vi "NPC3SG Live Control v10.6.2.vi"(1 "Running":refnum<vi>, 2 "Calibration File":path, 3 "Drive Live Controls":T1={"Snapshot"=FALSE, "Move Step"=0.5, "Move Home"=FALSE, "Move Down"=FALSE, "Move Up"=FALSE, "Move Left"=FALSE, "Move Right"=FALSE, "Move Out"=FALSE, "Move In"=FALSE} {"Move Step" min=0.0 max=30.0 step=0.1 format="%.3f"}, 4 "Drive Visa Name":refnum<visa-resource-name>="COM5") -> (0 "Reset Switches":bool)   [LabVIEW 2010]
uses:
  TypeDefs/NPC3SG Live Controls.ctl
panel:
  in  "Home":dbl=10.0 format="%.3f"
  # "XY"
  # "Z"
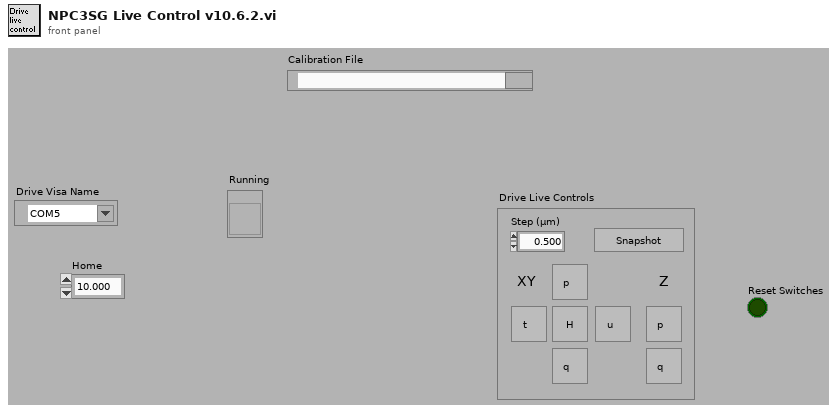
[diagram p1: front panel]
types:
  T1 = typedef "NPC3SG Live Controls.ctl" = cluster{"Snapshot":bool, "Move Step":dbl, "Move Home":bool, "Move Down":bool, "Move Up":bool, "Move Left":bool, "Move Right":bool, "Move Out":bool, "Move In":bool}
  T2 = typedef "NPC3SG Current Values.ctl" = cluster{"Drive X Position":dbl, "Drive Y Position":dbl, "Drive Z Position":dbl}
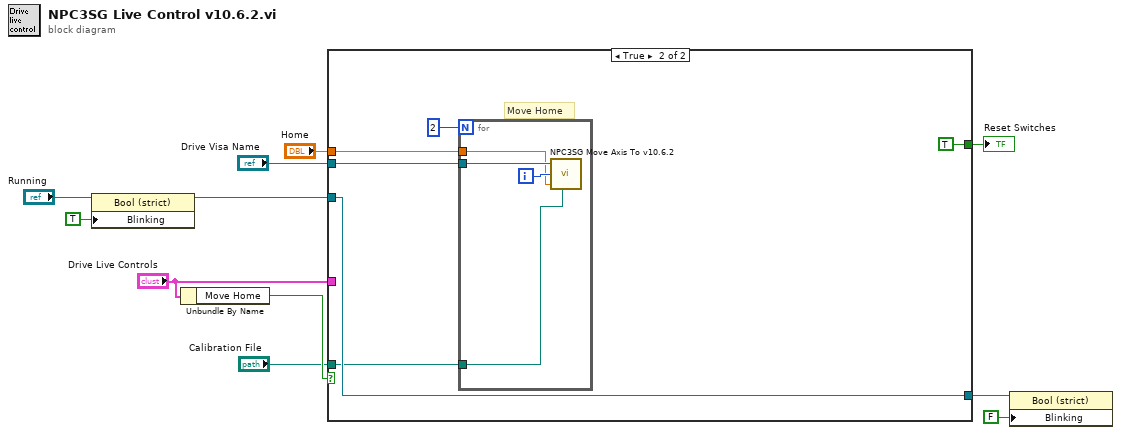
[diagram p0: block diagram]
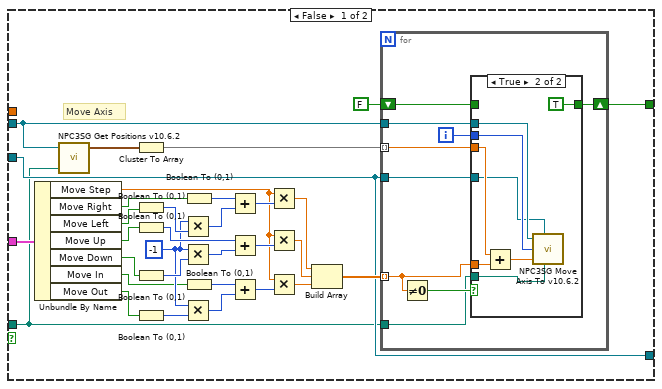
[diagram p2: hidden frame]
diagram:
  n1 = property class="Bool (strict)"(reference="Running", "Blinking"=TRUE ("Blinkend")) -> (reference out=w4:refnum<vi>)  [unwired: 1 in, 1 out]
  n2 = Unbundle By Name("Drive Live Controls") -> ("Move Home"=w9:bool)
  n3 = case shown="True" w9 {
    tunnel: "Drive Visa Name" -> [w18 w66]
    tunnel: [w16 TRUE ("Reset Switches")] -> w11
    tunnel: w4 -> [w14 w64]
    tunnel: "Drive Live Controls" -> [w19 _]
    tunnel: "Home" -> [_ w65]
    tunnel: [w14 w64] -> w2
    tunnel: "Calibration File" -> [w12 w62]
    frame False {
      w31 = -1
      # "Move Axis"
      n4 = Unbundle By Name(w19) -> ("Move Step"=w20:dbl, "Move Right"=w21:bool, "Move Left"=w26:bool, "Move Up"=w25:bool, "Move Down"=w24:bool, "Move In"=w23:bool, "Move Out"=w22:bool)
      n5 = call "NPC3SG Get Positions v10.6.2.vi"("Drive Visa Name"=w18, "Calibration File"=w12) -> ("Drive Current Values"=w13:T2)  [unwired: 5 in]
      n6 = Cluster To Array(cluster=w13) -> (array=w17:dbl[])
      n7 = Boolean To (0,1)(Boolean=w26) -> (0, 1=w33:i16)
      n8 = Boolean To (0,1)(Boolean=w25) -> (0, 1=w37:i16)
      n9 = Boolean To (0,1)(Boolean=w24) -> (0, 1=w34:i16)
      n10 = Boolean To (0,1)(Boolean=w22) -> (0, 1=w32:i16)
      n11 = Multiply(x=w31, y=w33) -> (x*y=w36:i32)
      n12 = Multiply(x=w31, y=w34) -> (x*y=w38:i32)
      n13 = Multiply(x=w31, y=w32) -> (x*y=w30:i32)
      n14 = Boolean To (0,1)(Boolean=w21) -> (0, 1=w35:i16)
      n15 = Boolean To (0,1)(Boolean=w23) -> (0, 1=w29:i16)
      n16 = Add(x=w35, y=w36) -> (x+y=w39:i32)
      n17 = Add(x=w37, y=w38) -> (x+y=w40:i32)
      n18 = Add(x=w29, y=w30) -> (x+y=w28:i32)
      n19 = Multiply(x=w20, y=w39) -> (x*y=w41:dbl)
      n20 = Multiply(x=w20, y=w40) -> (x*y=w42:dbl)
      n21 = Multiply(x=w20, y=w28) -> (x*y=w27:dbl)
      n22 = Build Array(w41, w42, w27) -> (w43:dbl[])
      n23 = for {
        tunnel: w43 -> [w51] mode=indexing
        tunnel: w18 -> [w52]
        tunnel: w17 -> [w46] mode=indexing
        shift-right: [w48] -> w16
        shift-left: FALSE ("Reset Switches") -> [w47]
        tunnel: w14 -> [w45]
        tunnel: w12 -> [w44]
        i -> [w49]
        n24 = Not Equal To 0?(x=w51) -> (x != 0?=w50:bool)
        n25 = case shown="True" w50 {
          tunnel: w51 -> [_ w58]
          tunnel: w52 -> [_ w61]
          tunnel: w49 -> [_ w60]
          tunnel: [w53 TRUE ("Reset Switches")] -> w48
          tunnel: w47 -> [w53 _]
          tunnel: w46 -> [_ w57]
          tunnel: w45 -> [_ w55]
          tunnel: w44 -> [_ w54]
          frame False {
          }
          frame True {
            n26 = Add(x=w57, y=w58) -> (x+y=w56:dbl)
            n27 = call "NPC3SG Move Axis To v10.6.2.vi"("Drive Visa Name"=w61, "Running"=w55, "Axis"=w60, "Drive Set"=w56, "Calibration File"=w54) -> ()  [unwired: 2 in, 1 out]
          }
        }
      }
    }
    frame True {
      # "Move Home"
      n28 = for {
        N: 2 -> [_]
        tunnel: w66 -> [w71]
        tunnel: w65 -> [w69]
        tunnel: w62 -> [w68]
        i -> [w70]
        n29 = call "NPC3SG Move Axis To v10.6.2.vi"("Drive Visa Name"=w71, "Axis"=w70, "Drive Set"=w69, "Calibration File"=w68) -> ()  [unwired: 3 in, 1 out]
      }
    }
  }
  "Reset Switches" <- w11
  n30 = property class="Bool (strict)"(reference=w2, "Blinking"=FALSE ("Blinkend")) -> ()  [unwired: 1 in, 2 out]
